vi "movearray to round conti move.vi"(1 "Position in":T1, 2 "move array":T3) -> (0 "move array out":T2)   [LabVIEW 2019]
uses:
  move array and radius.ctl
  move array.ctl
  position cluster.ctl
panel:
  out "radius":dbl
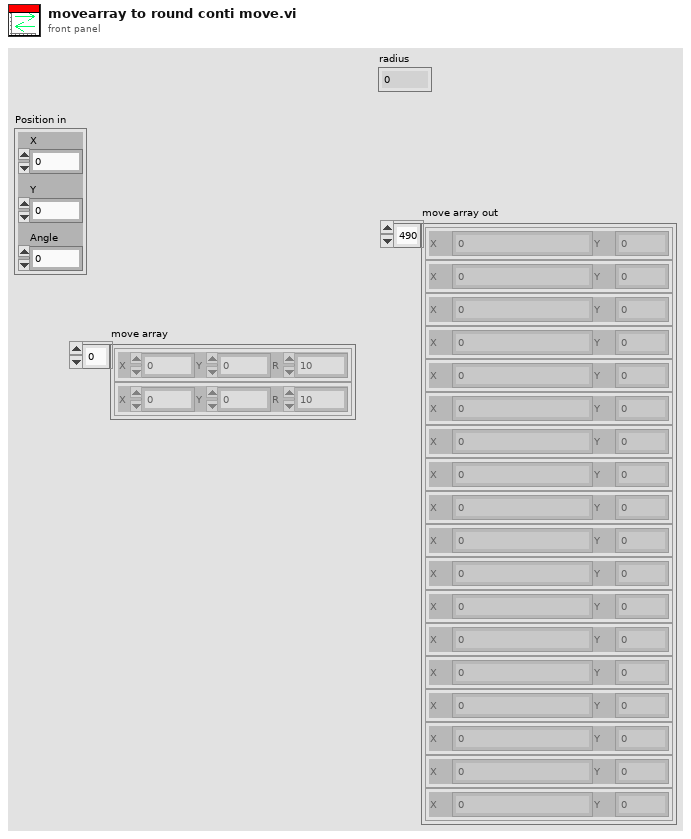
[diagram p1: front panel]
types:
  T1 = typedef "position cluster.ctl" = cluster{"X":dbl, "Y":dbl, "Angle":dbl}
  T2 = typedef "move array.ctl" = cluster{"X":dbl, "Y":dbl}[]
  T3 = typedef "move array and radius.ctl" = cluster{"X":dbl, "Y":dbl, "R":dbl}[]
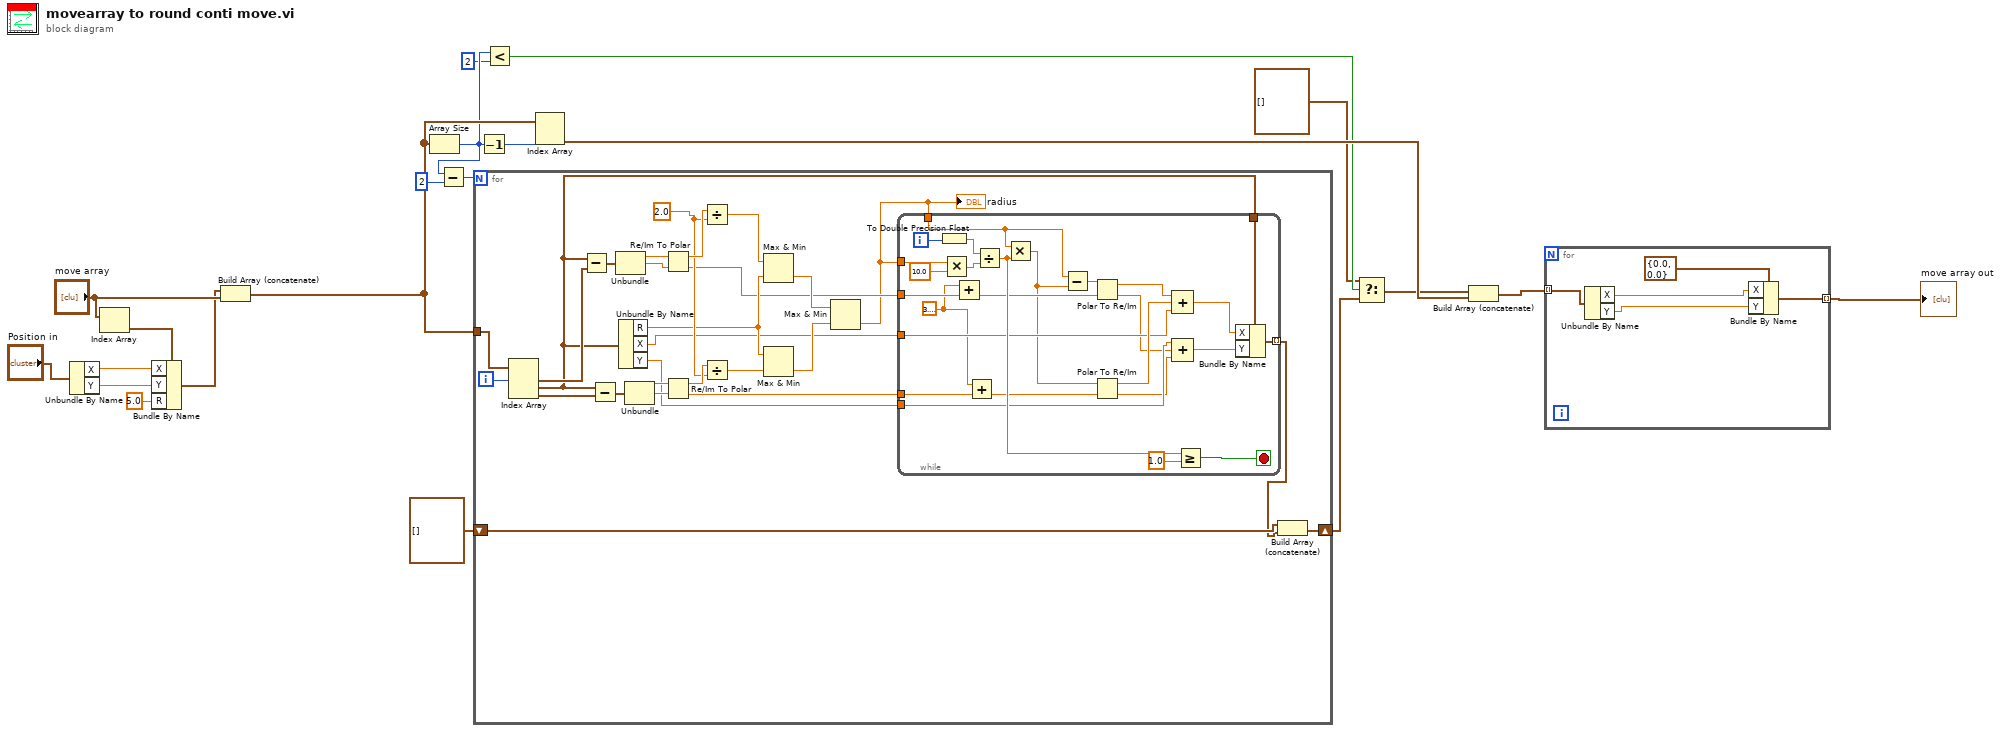
[diagram p0: block diagram]
diagram:
  n1 = Unbundle By Name("Position in") -> ("X"=w10:dbl, "Y"=w9:dbl)
  n2 = Index Array(array="move array") -> (element=w11:cluster{"X":dbl, "Y":dbl, "R":dbl})  [unwired: 1 in]
  n3 = Bundle By Name(cluster=w11, "X"=w10, "Y"=w9, "R"=5.0) -> (w8:cluster{"X":dbl, "Y":dbl, "R":dbl})
  n4 = Build Array (concatenate)(w8, "move array") -> (w14:T3)
  n5 = Array Size(array=w14) -> (size(s)=w6:i32)
  n6 = Subtract(x=w6, y=2) -> (x-y=w19:i32)
  n7 = for {
    N: w19 -> [_]
    tunnel: w14 -> [w47]
    shift-right: [w24] -> w3
    shift-left: cluster{"X":dbl, "Y":dbl, "R":dbl}[] [] -> [w23]
    i -> [w48]
    w35 = 2.0 ("y")
    n8 = Index Array(array=w47, index #1=w48) -> (element #1=w45:cluster{"X":dbl, "Y":dbl, "R":dbl}, element #2=w25:cluster{"X":dbl, "Y":dbl, "R":dbl}, element #3=w46:cluster{"X":dbl, "Y":dbl, "R":dbl})  [unwired: 2 in]
    n9 = Subtract(x=w25, y=w45) -> (x-y=w44:cluster{"X":dbl, "Y":dbl, "R":dbl})
    n10 = Subtract(x=w25, y=w46) -> (x-y=w41:cluster{"X":dbl, "Y":dbl, "R":dbl})
    n11 = Unbundle(w44) -> ("X"=w43:dbl, "Y"=w42:dbl)  [unwired: 1 out]
    n12 = Unbundle By Name(w25) -> ("R"=w34:dbl, "X"=w27:dbl, "Y"=w26:dbl)
    n13 = Unbundle(w41) -> ("X"=w39:dbl, "Y"=w40:dbl)  [unwired: 1 out]
    n14 = Re/Im To Polar(2:w42, 3:w43) -> (0:w30:dbl, 1:w38:dbl)
    n15 = Re/Im To Polar(2:w40, 3:w39) -> (0:w28:dbl, 1:w36:dbl)
    n16 = Divide(x=w38, y=w35) -> (x/y=w37:dbl)
    n17 = Divide(x=w36, y=w35) -> (x/y=w33:dbl)
    n18 = Max & Min(x=w37, y=w34) -> (min(x,y)=w31:dbl)  [unwired: 1 out]
    n19 = Max & Min(x=w34, y=w33) -> (min(x,y)=w32:dbl)  [unwired: 1 out]
    n20 = Max & Min(x=w31, y=w32) -> (min(x,y)=w29:dbl)  [unwired: 1 out]
    "radius" <- w29
    n21 = while {
      tunnel: w30 -> [w55]
      tunnel: w29 -> [w72]
      tunnel: w29 -> [w53]
      tunnel: w28 -> [w66]
      tunnel: w27 -> [w64]
      tunnel: w26 -> [w63]
      tunnel: w25 -> [w62]
      tunnel: [w59] -> w22 mode=indexing
      i -> [w73]
      stop <- w69 stop-if-true
      w50 = 3.141592653589793
      n22 = To Double Precision Float(number=w73) -> (double precision float=w74:dbl)
      n23 = Multiply(x=w72, y=10.0) -> (x*y=w70:dbl)
      n24 = Add(x=w50, y=w55) -> (x+y=w52:dbl)
      n25 = Add(x=w50, y=w66) -> (x+y=w51:dbl)
      n26 = Divide(x=w74, y=w70) -> (x/y=w68:dbl)
      n27 = Multiply(x=w53, y=w68) -> (x*y=w49:dbl)
      n28 = Subtract(x=w53, y=w49) -> (x-y=w54:dbl)
      n29 = Polar To Re/Im(2:w52, 3:w54) -> (0:w57:dbl, 1:w56:dbl)
      n30 = Polar To Re/Im(2:w51, 3:w49) -> (0:w58:dbl, 1:w65:dbl)
      n31 = Compound Arithmetic op=ADD(w56, w65, w64) -> (w61:dbl)
      n32 = Compound Arithmetic op=ADD(w63, w57, w58) -> (w60:dbl)
      n33 = Greater Or Equal?(x=w68, y=1.0) -> (x >= y?=w69:bool)
      n34 = Bundle By Name(cluster=w62, "X"=w61, "Y"=w60) -> (w59:cluster{"X":dbl, "Y":dbl, "R":dbl})
    }
    n35 = Build Array (concatenate)(w23, w22) -> (w24:cluster{"X":dbl, "Y":dbl, "R":dbl}[])
  }
  n36 = Decrement(x=w6) -> (x-1=w21:i32)
  n37 = Less?(x=w6, y=2) -> (x < y?=w2:bool)
  n38 = Index Array(array=w14, index #2=w21) -> (element #2=w20:cluster{"X":dbl, "Y":dbl, "R":dbl})  [unwired: 1 in, 1 out]
  n39 = Select(t=cluster{"X":dbl, "Y":dbl, "R":dbl}[] [], s=w2, f=w3) -> (s? t:f=w4:cluster{"X":dbl, "Y":dbl, "R":dbl}[])
  n40 = Build Array (concatenate)(w4, w20) -> (w17:cluster{"X":dbl, "Y":dbl, "R":dbl}[])
  n41 = for {
    tunnel: w17 -> [w79] mode=indexing
    tunnel: [w75] -> w16 mode=indexing
    n42 = Unbundle By Name(w79) -> ("X"=w77:dbl, "Y"=w76:dbl)
    n43 = Bundle By Name(cluster=cluster{"X":dbl, "Y":dbl} {"X"=0.0, "Y"=0.0} ("Cluster"), "X"=w77, "Y"=w76) -> (w75:cluster{"X":dbl, "Y":dbl})
  }
  "move array out" <- w16
